vi "Reset.vi"(8 "error in (no error)":errorcluster, 11 "VISA resource name":refnum<visa-resource-name>) -> (0 "error out":errorcluster, 3 "VISA resource name out":refnum<visa-resource-name>)   [LabVIEW 2022 SP3, in "Agilent E364X Series.lvlib"]
doc: "This VI resets the instrument. Consult the user's manual for the default parameter settings to which this command resets the instrument."
uses:
  Agilent E364X Series.lvlib
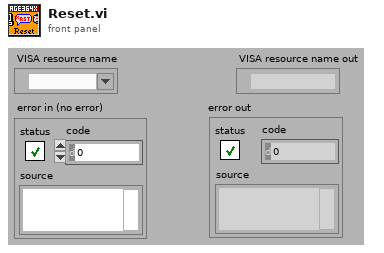
[diagram p1: front panel]
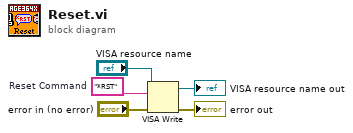
[diagram p0: block diagram]
diagram:
  w5 = "*RST"  # Reset Command
  n1 = VISA Write(VISA resource name="VISA resource name", write buffer=w5, error in (no error)="error in (no error)") -> (VISA resource name out=→"VISA resource name out":refnum<visa-resource-name>, error out=→"error out":errorcluster)  [unwired: 1 out]
